vi "Close Data File.vi"(8 "error in (no error)":errorcluster, 11 "File Ref":refnum<k20>) -> (0 "error out":errorcluster)   [LabVIEW 2015, in "Data Replay File.lvlib"]
uses:
  Data Replay File.lvlib
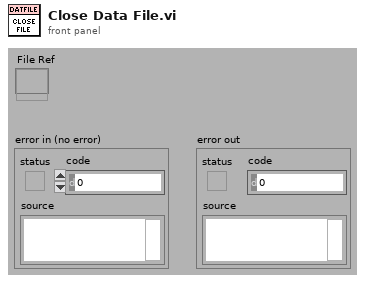
[diagram p1: front panel]
types:
  T1 = enum16{"UPDATE", "READ", "QUERY", "CREATE CHILD", "CREATE", "CONNECT", "DISCONNECT"}
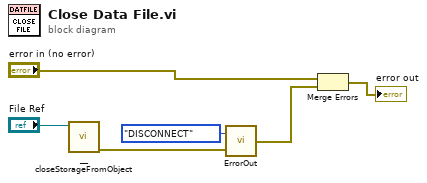
[diagram p0: block diagram]
diagram:
  n1 = call <vilib>:"__closeStorageFromObject.vi"("storage refnum"="File Ref") -> ("error out"=w2:errorcluster)  [unwired: 6 in]
  n2 = call <vilib>:"ErrorOut.vi"("error in"=w2, "DNL_NodeType"=T1."DISCONNECT") -> ("error out"=w1:errorcluster)
  n3 = Merge Errors("error in (no error)", w1) -> (→"error out":errorcluster)
